vi "Read in XW map for PolySurf_PN.vi"(0 "XW map file path (dialog if empty)":path=path "C:/Documents and Settings/Paul Nathan/Desktop/XW Calib Map/XW Calib Map POLYSURF vi/XW_Map_Wire001OH65_080210.txt") -> (1 "XW map values":dbl[][](array[numeric])=[[-45.0, 1.800895, 1.830505, 0.5789, 19.6], [-40.05, 1.801655, 1.830085, 0.5362, 19.6], [-34.92, 1.80276, 1.82851, 0.5637, 19.6], [-29.79, 1.80447, 1.826445, 0.5509, 19.6], [-25.02, 1.80642, 1.823675, 0.549, 19.6], [-20.25, 1.80957, 1.82, 0.5656, 19.6], [-15.12, 1.812855, 1.814825, 0.579, 19.6], [-9.81, 1.81675, 1.80899, 0.5538, 19.6], [-5.04, 1.821215, 1.80376, 0.528, 19.6], [0.0, 1.825705, 1.798205, 0.5414, 19.6], [4.86, 1.83083, 1.79222, 0.5426, 19.6], [10.08, 1.83678, 1.787235, 0.5731, 19.6], [15.21, 1.84271, 1.783015, 0.5721, 19.6], [19.71, 1.847695, 1.78017, 0.572, 19.6], [25.02, 1.85216, 1.77708, 0.5789, 19.6], [29.97, 1.85599, 1.774675, 0.5531, 19.6], [35.19, 1.859215, 1.773055, 0.5483, 19.6], [39.96, 1.86082, 1.77186, 0.5626, 19.6], [45.0, 1.86222, 1.77134, 0.5396, 19.6], [-45.0, 1.83518, 1.90668, 1.0167, 19.6], [-40.05, 1.83793, 1.90682, 1.0018, 19.6], [-34.92, 1.841365, 1.90547, 1.0258, 19.6], [-29.79, 1.84519, 1.901525, 1.0071, 19.6], [-25.02, 1.84992, 1.898115, 0.9934, 19.6], [-20.25, 1.85634, 1.892835, 1.002, 19.6], [-15.03, 1.86491, 1.887765, 0.9991, 19.6], [-9.81, 1.873695, 1.88023, 0.9975, 19.6], [-5.04, 1.881815, 1.87232, 1.0042, 19.6], [0.0, 1.889865, 1.864295, 0.9965, 19.6], [4.86, 1.89887, 1.85534, 1.0004, 19.6], [10.08, 1.907215, 1.846415, 1.0006, 19.6], [15.21, 1.914965, 1.837775, 0.9903, 19.6], [19.71, 1.921445, 1.830735, 1.003, 19.6], [24.75, 1.926975, 1.82336, 0.998, 19.6], [29.88, 1.93148, 1.8171, 1.0067, 19.6], [35.01, 1.934305, 1.811725, 1.0007, 19.6], [39.96, 1.936615, 1.80842, 1.0008, 19.6], [45.0, 1.937555, 1.80567, 1.0036, 19.6], [-45.0, 1.88892, 2.02289, 2.0085, 19.6], [-40.14, 1.894505, 2.02194, 1.9942, 19.7], [-34.92, 1.902435, 2.02069, 1.9997, 19.7], [-29.79, 1.913225, 2.01791, 2.0039, 19.7], [-25.29, 1.92448, 2.01374, 1.9963, 19.9], [-20.25, 1.9398, 2.008215, 2.0072, 19.9], [-15.12, 1.95598, 2.00029, 2.0067, 19.9], [-10.08, 1.972285, 1.99043, 1.9991, 19.8], [-5.04, 1.986135, 1.979965, 1.9999, 19.8], [0.0, 1.99866, 1.96829, 1.9949, 19.9], [4.86, 2.011405, 1.954655, 2.0035, 19.9], [10.08, 2.023045, 1.939745, 2.0038, 19.9], [15.21, 2.032605, 1.92335, 1.9981, 20.0], [19.71, 2.03973, 1.90924, 2.0028, 19.9], [24.75, 2.04603, 1.894395, 1.9971, 19.9], [29.97, 2.05053, 1.88109, 1.9993, 20.0], [35.19, 2.053585, 1.870395, 1.9998, 19.9], [39.96, 2.055075, 1.86296, 1.9936, 19.8], [45.0, 2.055295, 1.857395, 1.9996, 19.8], [-45.0, 1.933145, 2.106385, 3.0062, 19.9], [-40.05, 1.940805, 2.106315, 3.001, 19.9], [-34.92, 1.951665, 2.104905, 3.0056, 19.9], [-29.79, 1.96578, 2.10068, 2.9968, 20.0], [-25.02, 1.98216, 2.096465, 3.0032, 20.0], [-20.25, 2.00179, 2.0892515, 2.9922, 20.0], [-15.03, 2.023705, 2.08071775, 2.9993, 19.9], [-9.81, 2.045075, 2.06995, 3.0006, 19.9], [-5.04, 2.062425, 2.057735, 2.9992, 20.0], [0.0, 2.07712, 2.04351, 2.9915, 20.1], [4.86, 2.092355, 2.027415, 3.0019, 20.1], [10.08, 2.105585, 2.008005, 3.0045, 20.1], [15.21, 2.115655, 1.98684, 2.9996, 20.1], [19.71, 2.12358, 1.968255, 3.0044, 20.1], [24.75, 2.1296625, 1.94711, 2.9952, 20.1], [29.88, 2.1350495, 1.92924, 2.9962, 20.1], [35.19, 2.1388512, 1.91453, 3.0039, 20.1], [39.96, 2.14032625, 1.90473, 2.9987, 20.1], [45.0, 2.1402735, 1.89754, 3.0062, 20.1], [-45.0, 1.97018, 2.17184, 3.989, 20.1], [-40.05, 1.9782, 2.1723, 3.9975, 20.1], [-34.92, 1.990395, 2.170605, 3.9983, 20.1], [-29.79, 2.00819, 2.166705, 3.9926, 20.1], [-25.29, 2.028065, 2.16221, 4.0035, 20.1], [-19.89, 2.05278, 2.15473, 4.007, 20.1], [-15.03, 2.077645, 2.144655, 3.9967, 20.1], [-9.81, 2.101825, 2.132215, 3.9917, 20.1], [-5.04, 2.12239, 2.119945, 4.0037, 20.1], [0.0, 2.1396196, 2.104965, 4.0049, 20.1], [4.86, 2.1553315, 2.0853675, 3.9973, 20.0], [10.08, 2.169095, 2.06319, 3.9945, 20.0], [15.03, 2.180985, 2.039205, 4.0037, 20.0], [19.71, 2.189315, 2.016835, 4.001, 20.0], [24.75, 2.196635, 1.99182, 4.0035, 20.0], [29.88, 2.201875, 1.969095, 4.0013, 20.1], [35.01, 2.20525, 1.95105, 3.996, 20.1], [39.96, 2.20685, 1.939715, 3.9959, 20.1], [45.0, 2.206975, 1.93236, 4.0042, 20.1], [-45.0, 2.00413, 2.228735, 5.0015, 20.1], [-40.05, 2.01118, 2.228915, 5.0012, 20.1], [-34.92, 2.02463, 2.226635, 4.9979, 20.1], [-30.06, 2.04525, 2.222565, 5.0011, 20.1], [-25.29, 2.06769, 2.217195, 4.9987, 20.0], [-20.25, 2.0951, 2.20911, 4.9968, 20.0], [-15.03, 2.123315, 2.198695, 4.9981, 20.0], [-10.08, 2.1503775, 2.18576, 4.997, 20.0], [-5.04, 2.17222, 2.1717, 4.998, 20.1], [0.0, 2.191345, 2.155695, 5.0025, 20.1], [4.86, 2.20905, 2.135, 5.0092, 20.1], [10.08, 2.22319, 2.110085, 4.9984, 20.1], [15.21, 2.235495, 2.083186, 5.0029, 20.1], [19.71, 2.244165, 2.058005, 4.9987, 20.0], [25.02, 2.252215, 2.02966, 5.0007, 20.0], [29.88, 2.25803, 2.00352, 5.0008, 20.0], [35.19, 2.261635, 1.982405, 4.9969, 20.1], [39.96, 2.263275, 1.970055, 4.9981, 20.1], [45.0, 2.26317, 1.9631, 5.003, 20.1], [-45.0, 2.058, 2.320555, 7.0007, 20.1], [-40.05, 2.06419, 2.320555, 6.996, 20.1], [-34.92, 2.08087, 2.318335, 6.9966, 20.1], [-29.61, 2.10723, 2.31403, 7.0076, 20.1], [-25.29, 2.1340865, 2.30767, 6.997, 20.1], [-20.25, 2.166745, 2.298345, 6.9902, 20.1], [-15.03, 2.19938, 2.28731, 7.0039, 20.1], [-9.81, 2.23019, 2.272795, 7.0031, 20.1], [-5.04, 2.25453, 2.257245, 7.0001, 20.1], [0.0, 2.275755, 2.2388, 6.9961, 20.1], [4.86, 2.295475, 2.215345, 7.0049, 20.1], [10.08, 2.311685, 2.18721, 6.9991, 20.1], [15.03, 2.325015, 2.156335, 7.0029, 20.1], [19.71, 2.33442, 2.126925, 6.9944, 20.1], [24.75, 2.343575, 2.0933805, 7.0014, 20.1], [29.97, 2.35009, 2.060775, 7.0041, 20.1], [35.19, 2.35432, 2.03418, 7.0083, 20.1], [39.96, 2.355545, 2.019065, 6.9972, 20.1], [45.0, 2.35511, 2.013025, 6.9958, 20.1], [-45.0, 2.09865, 2.39536, 8.9926, 20.1], [-40.05, 2.10547, 2.39524, 8.9825, 20.1], [-34.92, 2.1262735, 2.393355, 9.0001, 20.1], [-29.79, 2.15808, 2.389085, 9.028, 20.1], [-25.29, 2.18864, 2.3813, 8.9917, 20.1], [-20.25, 2.22539, 2.3721, 9.0088, 20.1], [-15.03, 2.261505, 2.35982, 9.0168, 20.1], [-9.81, 2.293955, 2.343055, 8.9847, 20.1], [-5.04, 2.320645, 2.325835, 8.9741, 20.1], [0.0, 2.34454, 2.306995, 9.0006, 20.1], [5.04, 2.36534, 2.280665, 8.9879, 20.1], [10.08, 2.384, 2.25096, 9.021, 20.1], [15.03, 2.397825, 2.216365, 9.0002, 20.1], [19.71, 2.408905, 2.184615, 9.0172, 20.1], [24.75, 2.4167, 2.14541, 8.9759, 20.1], [29.88, 2.42426, 2.10807, 8.9923, 20.1], [35.01, 2.428835, 2.0755235, 8.9948, 20.1], [39.96, 2.43081, 2.057055, 9.0015, 20.1], [45.0, 2.431635, 2.051435, 9.0313, 20.1], [-45.0, 2.13115, 2.460385, 11.029, 20.1], [-40.05, 2.13971215, 2.460145, 11.0141, 20.1], [-34.92, 2.16358, 2.45648, 10.9868, 20.1], [-29.97, 2.19943, 2.450805, 10.9793, 20.2], [-25.29, 2.235245, 2.444165, 10.9919, 20.2], [-20.25, 2.27548, 2.434425, 11.0147, 20.2], [-15.03, 2.31343, 2.420385, 10.9931, 20.1], [-10.08, 2.349155, 2.403745, 10.9896, 20.1], [-5.04, 2.378475, 2.386095, 11.0043, 20.1], [0.0, 2.40296, 2.365255, 11.0025, 20.1], [4.86, 2.426915, 2.338585, 11.0401, 20.1], [10.08, 2.44409, 2.30395, 10.9835, 20.1], [15.21, 2.460045, 2.2681, 11.0065, 20.1], [19.71, 2.471095, 2.233105, 11.0026, 20.1], [24.75, 2.481035, 2.1915, 11.0039, 20.1], [29.97, 2.48751, 2.148325, 10.9759, 20.1], [35.19, 2.4926, 2.11057, 10.9899, 20.1], [39.96, 2.494855, 2.0878445, 10.9946, 20.1], [45.0, 2.49433, 2.079896215, 10.9895, 20.1], [-45.0, 2.156525, 2.515915, 13.0042, 20.1], [-39.87, 2.168245, 2.51564, 12.9889, 20.1], [-34.92, 2.197255, 2.5128, 12.9938, 20.2], [-29.7, 2.238575, 2.507375, 13.0079, 20.2], [-25.29, 2.2765, 2.49938, 12.9834, 20.3], [-19.98, 2.32052, 2.48981, 13.043, 20.3], [-15.03, 2.360115, 2.47471, 12.9969, 20.3], [-9.81, 2.39763, 2.456845, 12.9832, 20.3], [-5.04, 2.42777, 2.43785, 12.9737, 20.3], [0.0, 2.45423, 2.4161, 12.9894, 20.3], [4.86, 2.478835, 2.387525, 13.0175, 20.3], [10.08, 2.4986, 2.352815, 13.0138, 20.3], [15.21, 2.514755, 2.31373, 13.009, 20.3], [19.71, 2.525525, 2.276645, 12.9871, 20.3], [25.11, 2.53702, 2.23236, 13.0232, 20.3], [29.97, 2.54369, 2.185175, 12.9869, 20.3], [35.01, 2.54878, 2.141585, 12.9826, 20.3], [39.96, 2.55116, 2.113585, 13.0029, 20.3], [45.0, 2.550915, 2.103145, 13.0075, 20.3], [-45.0, 2.17868, 2.565895, 15.0045, 20.3], [-40.05, 2.19247, 2.565895, 14.9976, 20.3], [-34.92, 2.226895, 2.562915, 14.9964, 20.3], [-29.79, 2.272245, 2.557015, 14.998, 20.3], [-25.29, 2.314085, 2.54986, 15.0173, 20.3], [-20.25, 2.358855, 2.53799, 15.0018, 20.3], [-15.03, 2.401635, 2.52317, 14.9901, 20.3], [-9.81, 2.440815, 2.50458, 14.9744, 20.3], [-5.04, 2.47311, 2.48548, 15.0021, 20.3], [0.0, 2.50023, 2.462475, 15.0098, 20.3], [5.04, 2.525645, 2.43191, 15.0127, 20.3], [10.08, 2.54597, 2.395525, 14.9987, 20.3], [15.21, 2.56268, 2.354615, 14.9901, 20.3], [19.98, 2.574755, 2.31574, 14.9906, 20.3], [24.75, 2.585795, 2.26904, 14.9989, 20.3], [29.88, 2.593995, 2.21821, 15.0041, 20.3], [35.1, 2.599595, 2.1698, 15.0142, 20.3], [39.96, 2.60106, 2.135825, 14.989, 20.3], [45.0, 2.601035, 2.122505, 15.0047, 20.3]], 2 "Zero angle dataset from map (used for calib. correction)":dbl[][](array[numeric])=[[1.825705, 1.798205, 0.5414, 19.6], [1.889865, 1.864295, 0.9965, 19.6], [1.99866, 1.96829, 1.9949, 19.9], [2.07712, 2.04351, 2.9915, 20.1], [2.1396196, 2.104965, 4.0049, 20.1], [2.191345, 2.155695, 5.0025, 20.1], [2.275755, 2.2388, 6.9961, 20.1], [2.34454, 2.306995, 9.0006, 20.1], [2.40296, 2.365255, 11.0025, 20.1], [2.45423, 2.4161, 12.9894, 20.3], [2.50023, 2.462475, 15.0098, 20.3]] format="%0.3f", 3 "XW map file path":path=path "C:/Documents and Settings/Paul Nathan/Desktop/XW Calib Map/XW Calib Map POLYSURF vi/XW_Map_Wire001OH65_080210.txt", 4 "pts per set":i32)   [LabVIEW 2011]
uses:
  <vilib>/Utility/file.llb/Read From Spreadsheet File (DBL).vi
  <vilib>/Utility/file.llb/Read From Spreadsheet File (string).vi
panel:
  # "Paul Nathan 17/02/10"
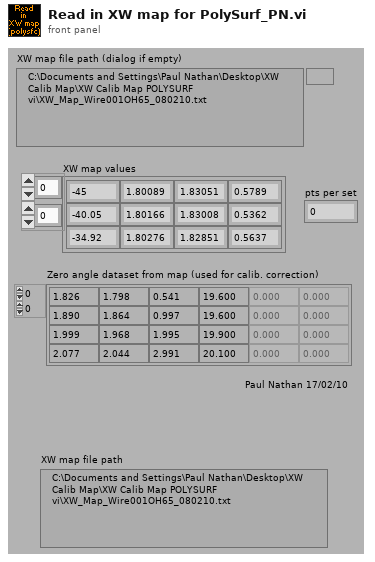
[diagram p1: front panel]
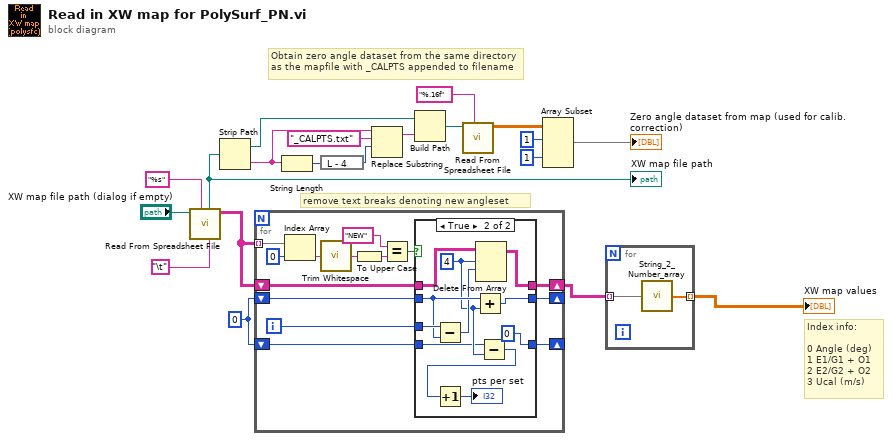
[diagram p0: block diagram]
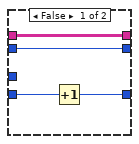
[diagram p2: hidden frame]
diagram:
  w1 = 0 ("length")
  # "remove text breaks denoting new angleset"
  # "Obtain zero angle dataset from the same directory as the mapfile with _CALPTS appended to filename"
  # "Index info:\n\n0 Angle (deg)\n1 E1/G1 + O1\n2 E2/G2 + O2\n3 Ucal (m/s)"
  n1 = call-poly <vilib>:"Read From Spreadsheet File.vi"("delimiter (\\t)"="\t", "format (%s)"="%s", "file path (dialog if empty)"="XW map file path (dialog if empty)") -> ("all rows"=w4:string[][], "new file path (Not A Path if cancelled)"=w6:path)  [unwired: 2 in, 5 out]
  "XW map file path" <- w6
  n2 = Strip Path(path=w6) -> (stripped path=w14:path, name=w18:string)
  n3 = for {
    tunnel: w4 -> [w34] mode=indexing
    shift-right: [w29] -> w3
    shift-left: w4 -> [w30]
    shift-right: [w27] -> _
    shift-left: w1 -> [w28]
    shift-right: [w21] -> _
    shift-left: w1 -> [w22]
    i -> [w26]
    n4 = Index Array(array=w34, index=0) -> (element=w25:string)
    n5 = call <vilib>:"Trim Whitespace.vi"("string"=w25) -> ("trimmed string"=w24:string)  [unwired: 1 in]
    n6 = To Upper Case(1:w24) -> (0:w23:string)
    n7 = Equal?(x="NEW" ("format (%s)"), y=w23) -> (x = y?=w31:bool)
    n8 = case shown="True" w31 {
      tunnel: w30 -> [w38 w49]
      tunnel: w28 -> [w37 w45]
      tunnel: [w38 w48] -> w29
      tunnel: [w37 w47] -> w27
      tunnel: w26 -> [_ w46]
      tunnel: w22 -> [w35 w42]
      tunnel: [w36 0] -> w21
      frame False {
        n9 = Increment(x=w35) -> (x+1=w36:i32)
      }
      frame True {
        w43 = 4 ("length")
        n10 = Subtract(x=w46, y=w45) -> (x-y=w44:i32)
        n11 = Add(x=w45, y=w43) -> (x+y=w47:i32)
        n12 = Delete From Array(array=w49, length=w43, index (row)=w44) -> (array with subset deleted=w48:string[][])  [unwired: 1 in, 1 out]
        n13 = Subtract(x=w42, y=w43) -> (x-y=w40:i32)
        n14 = Increment(x=w40) -> (x+1=→"pts per set":i32)
      }
    }
  }
  n15 = String Length(string=w18) -> (length=w17:i32)
  n16 = expression code="L - 4"(w17) -> (w16:i32)
  n17 = Replace Substring(3:w16, 4:"_CALPTS.txt" ("substring (\"\")"), 5:w18) -> (1:w13:string)  [unwired: 2 out]
  n18 = Build Path(base path=w14, name or relative path=w13) -> (appended path=w8:path)
  n19 = call-poly <vilib>:"Read From Spreadsheet File.vi"("format (%.3f)"="%.16f", "file path (dialog if empty)"=w8) -> ("all rows"=w10:dbl[][])  [unwired: 2 in, 7 out]
  n20 = Array Subset(array=w10, index (row)=1 ("index"), index (col)=1 ("index")) -> (→"Zero angle dataset from map (used for calib. correction)":dbl[][])  [unwired: 2 in]
  n21 = for {
    tunnel: w3 -> [w51] mode=indexing
    tunnel: [w50] -> w2 mode=indexing
    n22 = call "String_2_Number_array.vi"("Input String"=w51) -> ("Values"=w50:dbl[])
  }
  "XW map values" <- w2
